vi "Change Value.vi"(0 "String":string) -> (4 "String Out":string)   [LabVIEW 2021, in "InstrumentStudio Plug-In Editor.lvlib"]
uses:
  InstrumentStudio Plug-In Editor.lvlib
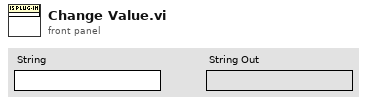
[diagram p1: front panel]
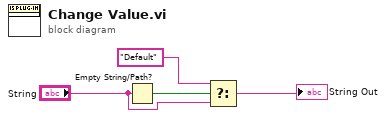
[diagram p0: block diagram]
diagram:
  n1 = Empty String/Path?(string/path="String") -> (empty?=w4:bool)
  n2 = Select(t="Default", s=w4, f="String") -> (s? t:f=→"String Out":string)
